vi "test Get and Set Iteration.vi"(8 "error in (no error)":errorcluster, 11 "TestCase in":refnum<class "Framework Property Tests.lvclass">) -> (0 "error out":errorcluster, 3 "TestCase out":refnum<class "Framework Property Tests.lvclass">)   [LabVIEW 2017, in "Framework Property Tests.lvclass"]
uses:
  Framework Property Tests.lvclass
  Mock Framework Class/Mock Framework.lvclass
  C:/github/data-sharing-framework/Data Sharing Framework Core/Engine/Classes/Framework/Framework.lvclass
  Engine/Classes/Framework/Framework.lvclass/Framework.ctl
  <vilib>/addons/_JKI Toolkits/VI Tester/TestCase.llb/TestCase.lvclass
  Engine/Classes/Framework/Framework.lvclass
  C:/Program Files (x86)/National Instruments/LabVIEW 2017/vi.lib/addons/_JKI Toolkits/VI Tester/TestCase.llb/TestCase.lvclass
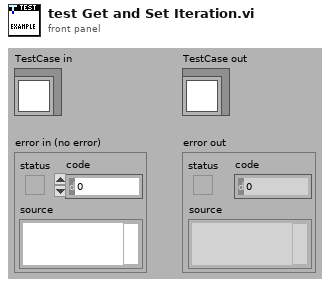
[diagram p1: front panel]
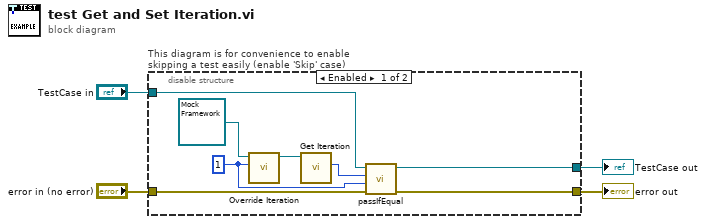
[diagram p0: block diagram]
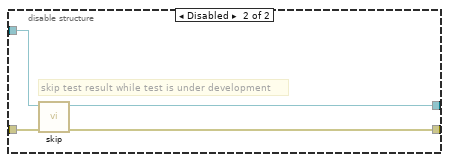
[diagram p2: hidden frame]
diagram:
  n1 = disable-structure "This diagram is for convenience to enable skipping a test easily (enable 'Skip' case)" shown="Enabled" {
    disable-tunnel: "TestCase in" -> [w10 w16]
    disable-tunnel: [w9 w14] -> w1
    disable-tunnel: [w11 w15] -> w2
    disable-tunnel: "error in (no error)" -> [w12 w13]
    frame Enabled {
      w6 = u64 1 ("iteration")
      n2 = call "Override Iteration.vi"("iteration"=w6, "Mock Framework in"=refnum<class "Mock Framework.lvclass"> refnum) -> ("Mock Framework out"=w8:refnum<class "Mock Framework.lvclass">)  [unwired: 8 in, 1 out]
      n3 = call "Get Iteration.vi"("Framework in"=w8) -> ("iteration"=w5:u64)  [unwired: 9 in, 1 out]
      n4 = call-dynamic "passIfEqual.vi"("error in (no error)"=w12, "y"=w6, "x"=w5, "TestCase in"=w10) -> ("error out"=w11:errorcluster, "TestCase out"=w9:refnum<class "Framework Property Tests.lvclass">)  [unwired: 6 in]
    }
    frame Disabled {
      # "skip test result while test is under development"
      n5 = call <vilib>:"skip.vi"("error in (no error)"=w13, "TestCase in"=w16) -> ("error out"=w15:errorcluster, "TestCase out"=w14:refnum<class "Framework Property Tests.lvclass">)  [unwired: 8 in]
    }
  }
  "error out" <- w2
  "TestCase out" <- w1
